vi "Extra_info.vi"() -> ()   [LabVIEW 2010]
panel:
  in  "Channel Names":string[](array[string])
  in  "Channel Values":string[](array[string])
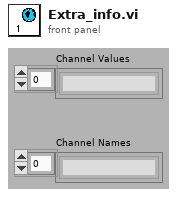
[diagram p1: front panel]
diagram:
